vi "AskForPlaylist.vi"(2 "Title":string="Enter a playlist name", 3 "Name":string) -> (0 "success":bool, 1 "name":string)   [LabVIEW 2012]
panel:
  in  "Cancel":bool
  in  "Ok":bool
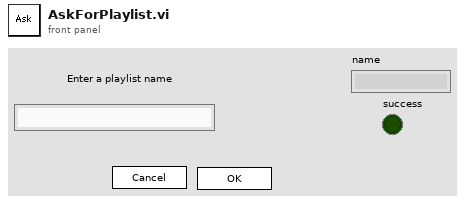
[diagram p1: front panel]
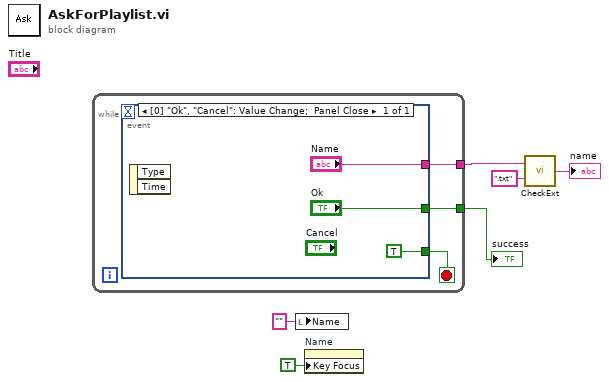
[diagram p0: block diagram]
diagram:
  n1 = while {
    tunnel: [w9] -> w4
    tunnel: [w8] -> w6
    stop <- w7 stop-if-true
    n2 = event shown="[0] \"Ok\", \"Cancel\": Value Change;  Panel Close" {
      selector: _ -> [_]
      dyn-events: _ -> [_]
      timeout: _ -> [_]
      tunnel: ["Name"] -> w9
      tunnel: ["Ok"] -> w8
      tunnel: [TRUE] -> w7
      event "Ok", "Cancel": Value Change; Panel Close {
        n3 = event-data() -> ()  [unwired: 1 in, 2 out]
      }
    }
  }
  "success" <- w6
  n4 = local write "Name"("" ("Name")) -> ()
  n5 = property on="Name" class="Str"("Key Focus"=TRUE) -> ()  [unwired: 2 in, 2 out]
  n6 = call "CheckExt.vi"("extension"=".txt" ("search string/char (-)"), "Name in"=w4) -> ("Name"=→"name":string)
